vi "ntr-init-io.vi"(11 "NutritionConfiguration":T1[](array[typedef]) {"ORP Dosing"."MIX Limit" format="%d [s]"; "ORP Dosing"."MIX Dose" format="%d [s]"; "PH Dosing"."ACID Limit" format="%d [s]"; "PH Dosing"."BASE Limit" format="%d [s]"; "PH Dosing"."ACID Dose" format="%d [s]"; "PH Dosing"."BASE Dose" format="%d [s]"; "EC Dosing"."BETA2 Limit" format="%d [s]"; "EC Dosing"."ALFA2 Limit" format="%d [s]"; "EC Dosing"."ALFA2 Dose" format="%d [s]"; "EC Dosing"."BETA2 Dose" format="%d [s]"; "EC Dosing"."BETA1 Limit" format="%d [s]"; "EC Dosing"."ALFA1 Limit" format="%d [s]"; "EC Dosing"."ALFA1 Dose" format="%d [s]"; "EC Dosing"."BETA1 Dose" format="%d [s]"; "Main"."DailyActivityHours"."Begin Time" format="ON:    %<%H:%M>T"; "Main"."DailyActivityHours"."End Time" format="OFF:    %<%H:%M>T"; "Main"."WashTimes"."Out" format="Wash out: %d [sec]"; "Main"."WashTimes"."In" format="Wash in: %d [sec]"; "Water Dosing"."Water Limit" format="%d [s]"; "Water Dosing"."Water Dose" format="%d [s]"}) -> (0 "error out":errorcluster)   [LabVIEW 2024]
uses:
  controls/UiNutritionPanel.ctl
  controls/UiScheduleTimestamp.ctl
  controls/eng-call-do-by-name.ctl
  controls/state-engine.ctl
  globals/globals-engine.vi
panel:
  # "Water"
  # "EC"
  # "PH"
  # "ORP"
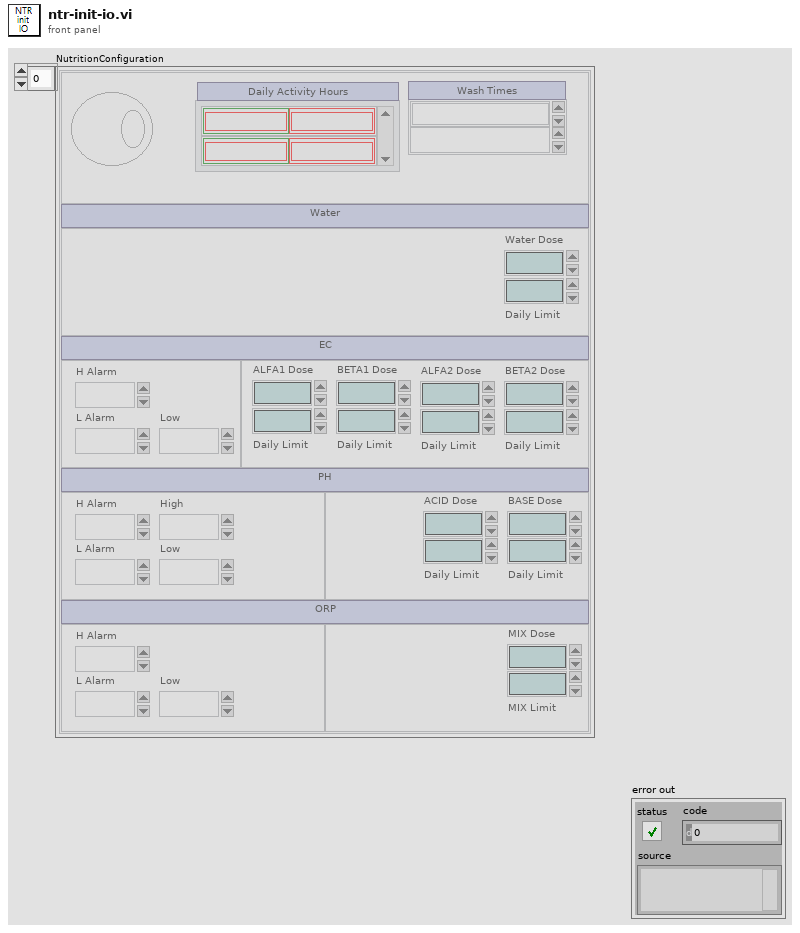
[diagram p1: front panel]
types:
  T1 = typedef "UiNutritionPanel.ctl" = cluster{"Main":cluster{"Enable":bool, "WashTimes":cluster{"In":dbl, "Out":dbl}, "DailyActivityHours":cluster{"Begin Time":T2, "End Time":T2}[]}, "Water Dosing":cluster{"Water Dose":dbl, "Water Limit":dbl}, "EC Ranges":cluster{"H Alarm":dbl, "L Alarm":dbl, "Low":dbl}, "EC Dosing":cluster{"ALFA1 Dose":dbl, "ALFA1 Limit":dbl, "BETA1 Dose":dbl, "BETA1 Limit":dbl, "ALFA2 Dose":dbl, "ALFA2 Limit":dbl, "BETA2 Dose":dbl, "BETA2 Limit":dbl}, "PH Ranges":cluster{"H Alarm":dbl, "L Alarm":dbl, "High":dbl, "Low":dbl}, "PH Dosing":cluster{"ACID Dose":dbl, "ACID Limit":dbl, "BASE Dose":dbl, "BASE Limit":dbl}, "ORP Ranges":cluster{"H Alarm":dbl, "L Alarm":dbl, "Low":dbl}, "ORP Dosing":cluster{"MIX Dose":dbl, "MIX Limit":dbl}}
  T2 = typedef "UiScheduleTimestamp.ctl" = timestamp
  T3 = typedef "eng-call-do-by-name.ctl" = cluster{"State":bool, "Timeout":u16, "Name":string}
  T4 = typedef "state-engine.ctl" = enum16{"ENG.NO-OP", "ENG.START", "ENG.STOP", "ENG.EXECUTE", "ENG.STATUS", "ENG.EXTERNAL-CALL", "ENG.INIT", "ENG.INIT.VARS", "ENG.INIT.SERIAL", "ENG.LOAD", "ENG.LOAD.SINGLE", "ENG.LOAD.MODULE", "ENG.LOAD.RELOAD", "ENG.LOAD.UNLOAD", "ENG.IO.LOAD", "ENG.IO.SAVE", "ENG.PROC.RELOAD-BY-NAME", "ENG.PROC.START", "ENG.PROC.STOP", "ENG.PROC.INSERT-STEPS", "ENG.PROC.ISRUNNING", "ENG.PROC.PRESET", "ENG.PROC.STATUS", "ENG.PRINT-USER-MSG", "ENG.RIO.SNAPSHOT", "ENG.RIO.AIN-SNAPSHOT-CALIB", "ENG.RIO.DOUT-BY-ADDR", "ENG.RIO.DOUT-BY-NAME", "ENG.RIO.RFS-DELAY-SET-X1", "ENG.RIO.RFS-DELAY-SET-X8", "ENG.RIO.RFS-CYCLES-SET", "ENG.RIO.RFS-CYCLES-GET", "ENG.RIO.RFS-ENABLE", "ENG.EXIT"}
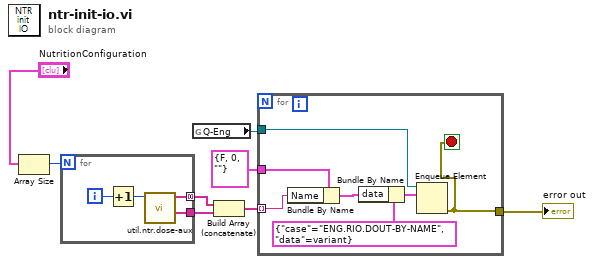
[diagram p0: block diagram]
diagram:
  n1 = Array Size(array="NutritionConfiguration") -> (size(s)=w5:i32)
  n2 = for {
    N: w5 -> [_]
    tunnel: [w10] -> w4 mode=concatenating
    tunnel: [w9] -> w3
    i -> [w12]
    n3 = Increment(x=w12) -> (x+1=w11:i32)
    n4 = call "util.ntr.dose-aux.vi"("Unit Index"=w11) -> ("DO Dose pumps"=w9:string[], "DO Unit Pumps"=w10:string[])  [unwired: 6 in, 3 out]
  }
  n5 = global read "globals-engine.vi" "Q-Eng"() -> (w1:refnum<queue>)
  n6 = Build Array (concatenate)(w4, w3) -> (w2:string[])
  n7 = for {
    tunnel: w2 -> [w18] mode=indexing
    tunnel: T3 {"State"=FALSE, "Timeout"=0, "Name"=""} ("Cluster") -> [w19]
    tunnel: w1 -> [w15]
    tunnel: [w13] -> w8
    stop <- w13 stop-if-true
    n8 = Bundle By Name(cluster=w19, "Name"=w18) -> (w14:T3)
    n9 = Bundle By Name(cluster=cluster{"case":T4, "data":variant} {"case"=enum."ENG.RIO.DOUT-BY-NAME", "data"=variant} ("element"), "data"=w14) -> (w16:cluster{"case":T4, "data":variant})
    n10 = Enqueue Element(queue=w15, element=w16) -> (error out=w13:errorcluster)  [unwired: 2 in, 2 out]
  }
  "error out" <- w8
